vi "OrderDeviceList.vi"(8 "error in (no error)":errorcluster, 10 "Slave Devices In":T1(array[cluster]), 11 "Device List In":refnum<class "Device.lvclass">[](array[class])) -> (0 "error out":errorcluster, 1 "Changes Made":bool, 2 "Slave Devices Out":T1(array[cluster]), 3 "Device List Out":refnum<class "Device.lvclass">[](array[class]))   [LabVIEW 2013]
uses:
  Device/Device.lvclass
  Pulseblaster/Pulseblaster.lvclass
  ColumnVIs/Column/Column.lvclass
  ColumnVIs/ModeCol/ModeCol.lvclass
  ColumnVIs/GroupCol/GroupCol.lvclass
  ColumnVIs/DigitalCol/DigitalCol.lvclass
  ColumnVIs/TriggerCol/TriggerCol.lvclass
  NI Card/NI Card.lvclass
  Slave_Pulseblaster/Slave_Pulseblaster.lvclass
panel:
  in  "Cancel Button":bool
  in  "OK Button":bool
  out "Master Name":string="Master Device"
  in  "Device Order":i32(listbox)
  # "WARNING: Changing device order destroys undo history"
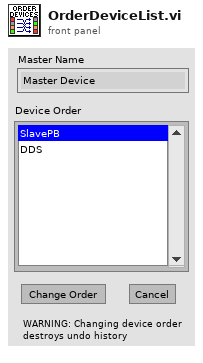
[diagram p1: front panel]
types:
  T1 = cluster{"Delete?":bool, "2D Picture":picture, "Name":string, "Edit Device":bool}[]
  T2 = cluster{"Delete?":bool, "2D Picture":picture, "Name":string, "Edit Device":bool}
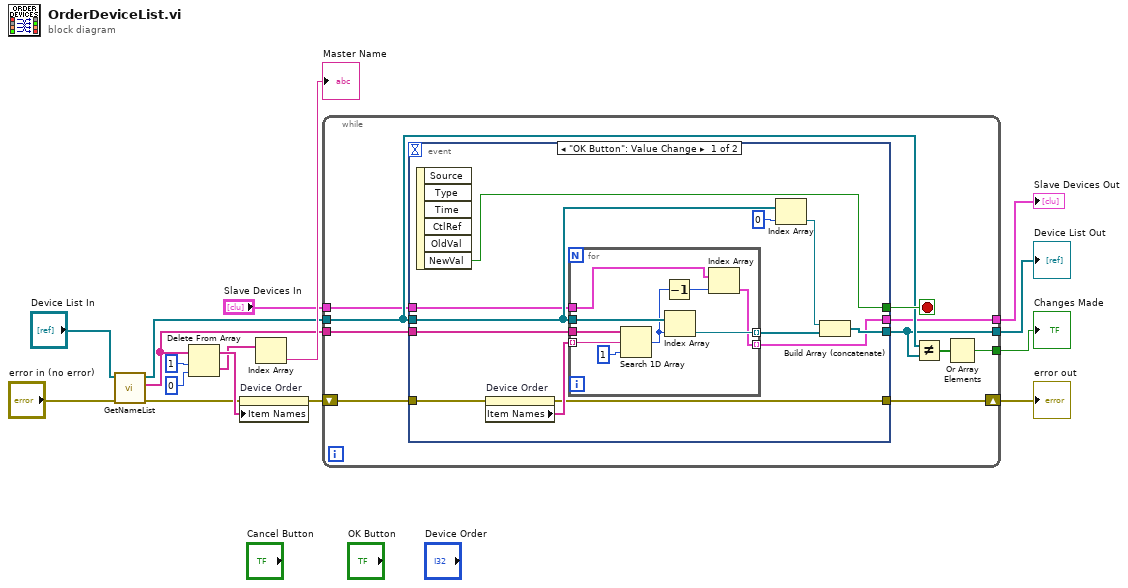
[diagram p0: block diagram]
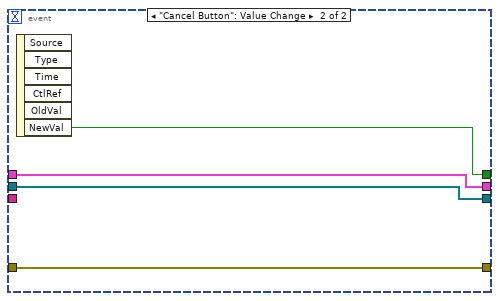
[diagram p2: hidden frame]
diagram:
  n1 = call "GetNameList.vi"("error in (no error)"="error in (no error)", "Devices"="Device List In") -> ("error out"=w8:errorcluster, "Names in use"=w11:string[], "Devices out"=w6:refnum<class "Device.lvclass">[])  [unwired: 7 in]
  n2 = Delete From Array(array=w11, length=1, index=0) -> (deleted portion=w13:string[], array with subset deleted=w15:string[])
  n3 = property on="Device Order" class="LstBox (strict)"(error in=w8, "Item Names"=w15) -> (error out=w7:errorcluster)  [unwired: 1 in, 1 out]
  n4 = Index Array(array=w13) -> (element=→"Master Name":string)  [unwired: 1 in]
  n5 = while {
    tunnel: w11 -> [w24]
    tunnel: [w23] -> w10
    shift-right: [w22] -> w3
    shift-left: w7 -> [w25]
    tunnel: w6 -> [w20]
    tunnel: [w19] -> w4
    tunnel: [w18] -> w2
    tunnel: "Slave Devices In" -> [w17]
    stop <- w26 stop-if-true
    n6 = event shown="[0] \"OK Button\": Value Change" {
      selector: _ -> [_ _]
      dyn-events: _ -> [_ _]
      timeout: _ -> [_ _]
      tunnel: [w27 w48] -> w26
      tunnel: w25 -> [w34 w51]
      tunnel: w24 -> [w35 _]
      tunnel: [w33 w50] -> w19
      tunnel: [w31 w51] -> w22
      tunnel: w20 -> [w30 w50]
      tunnel: [w29 w49] -> w18
      tunnel: w17 -> [w28 w49]
      event "OK Button": Value Change {
        n7 = event-data() -> ("NewVal"=w27:bool)  [unwired: 1 in, 5 out]
        n8 = property on="Device Order" class="LstBox (strict)"(error in=w34) -> (error out=w31:errorcluster, "Item Names"=w36:string[])  [unwired: 1 in, 1 out]
        n9 = for {
          tunnel: w36 -> [w47] mode=indexing
          tunnel: w35 -> [w46]
          tunnel: [w44] -> w32 mode=indexing
          tunnel: w30 -> [w43]
          tunnel: [w41] -> w29 mode=indexing
          tunnel: w28 -> [w42]
          n10 = Search 1D Array(1D array=w46, element=w47, start index (0)=1) -> (index of element=w39:i32)
          n11 = Decrement(x=w39) -> (x-1=w40:i32)
          n12 = Index Array(array=w43, index=w39) -> (element=w44:refnum<class "Device.lvclass">)
          n13 = Index Array(array=w42, index=w40) -> (element=w41:T2)
        }
        n14 = Index Array(array=w30, index=0) -> (element=w37:refnum<class "Device.lvclass">)
        n15 = Build Array (concatenate)(w37, w32) -> (w33:refnum<class "Device.lvclass">[])
      }
      event "Cancel Button": Value Change {
        n16 = event-data() -> ("NewVal"=w48:bool)  [unwired: 1 in, 5 out]
      }
    }
    n17 = Not Equal?(x=w20, y=w19) -> (x != y?=w21:bool[])
    n18 = Or Array Elements(Boolean array=w21) -> (logical OR=w23:bool)
  }
  "Device List Out" <- w4
  "Changes Made" <- w10
  "error out" <- w3
  "Slave Devices Out" <- w2
